vi "loadDATA.vi"() -> ()   [LabVIEW 2026]
panel:
  in  "dt":dbl
  out "Waveform Graph":waveform(dbl)(graph)
  out "channel name(s) out":string[](array[string])
  in  "file path":path
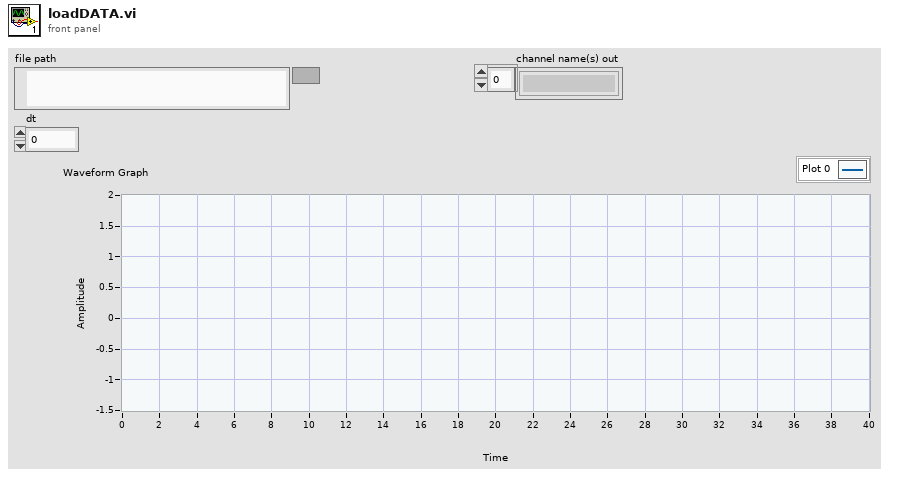
[diagram p1: front panel]
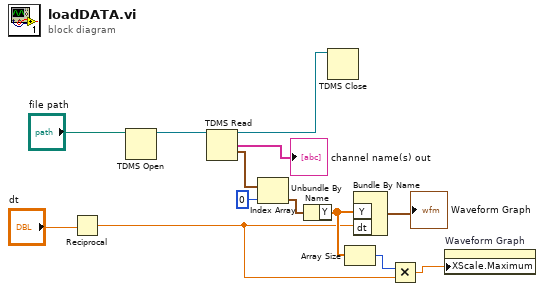
[diagram p0: block diagram]
diagram:
  n1 = Reciprocal(x="dt") -> (1/x=w2:dbl)
  n2 = TDMS Open(11:"file path") -> (3:w12:refnum<k34>)  [unwired: 6 in, 1 out]
  n3 = TDMS Read(0:w12) -> (4:w10:refnum<k34>, 8:→"channel name(s) out":string[], 10:w9:waveform(dbl)[])  [unwired: 7 in, 3 out]
  n4 = Index Array(array=w9, index=0) -> (element=w7:waveform(dbl))
  n5 = Unbundle By Name(w7) -> ("Y"=w4:dbl[])
  n6 = TDMS Close(11:w10) -> ()  [unwired: 1 in, 2 out]
  n7 = Array Size(array=w4) -> (size(s)=w3:i32)
  n8 = Bundle By Name("Y"=w4, "dt"=w2) -> (→"Waveform Graph":waveform(dbl))  [unwired: 1 in]
  n9 = Multiply(x=w3, y=w2) -> (x*y=w1:dbl)
  n10 = property on="Waveform Graph" class="WFGraph (strict)"("XScale.Maximum"=w1) -> ()  [unwired: 2 in, 2 out]
